vi "Tektonik.vi"() -> ()   [LabVIEW 2015]
uses:
  <vilib>/Utility/error.llb/DialogType.ctl
  <instrlib>/Tektronix TDS 200 1000 2000 Series/Public/Data/Read (Single Waveform).vi
  <vilib>/express/express analysis/Spectral/Block/exnSpectralBlock spectral measurements RMS poly.vi
  <vilib>/express/express analysis/Spectral/Block/exnSpectralBlock spectral measurements RMS WFM.vi
  <vilib>/express/express analysis/Spectral/XNode/ExpressSpectralMeasurementsBlockNode.xnode
  <instrlib>/Tektronix TDS 200 1000 2000 Series/Tektronix TDS 200 1000 2000 Series.lvlib
panel:
  out "Units 2":string
  out "Vpp":dbl
  out "FFT":cluster{"f0":dbl, "df":dbl, "magnitude":dbl[]}(graph)
  out "Units":string
  out "Freq":dbl
  in  "VISA resource name":refnum<visa-resource-name>
  in  "Serial Configuration":T1={"Baud Rate"=9600, "Parity"=0, "Stop Bits"=10, "Flow Control"=2} {"Flow Control" items=["None", "XON/XOFF", "RTS/CTS", "XON/XOFF & RTS/CTS", "DTR/DSR", "XON/XOFF & DTR/DSR"]; "Stop Bits" items=["1.0"=10, "1.5"=15, "2.0"=20]; "Parity" items=["None", "Odd", "Even", "Mark", "Space"]; "Baud Rate" items=["300"=300, "600"=600, "1200"=1200, "2400"=2400, "4800"=4800, "9600"=9600, "19200"=19200]}
  out "Waveform Graph":waveform(dbl)(graph)
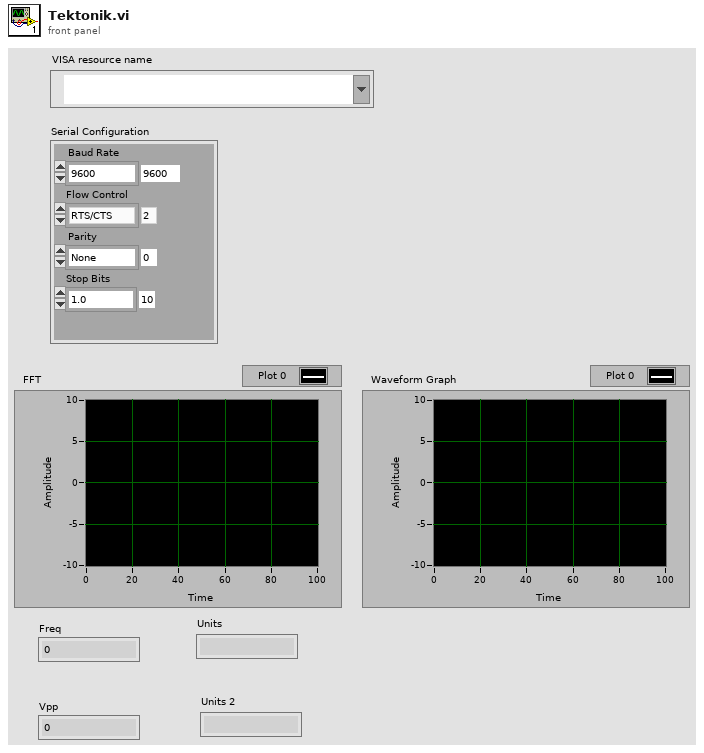
[diagram p1: front panel]
types:
  T1 = cluster{"Baud Rate":u32, "Parity":u16, "Stop Bits":u16, "Flow Control":u16}
  T2 = typedef "DialogType.ctl" = u16
  T3 = cluster{"averaging mode":u16, "weighting mode":u16, "number of averages":u32}
  T4 = cluster{"dB On (F)":bool, "unwrap phase (F)":bool, "convert to degree (F)":bool}
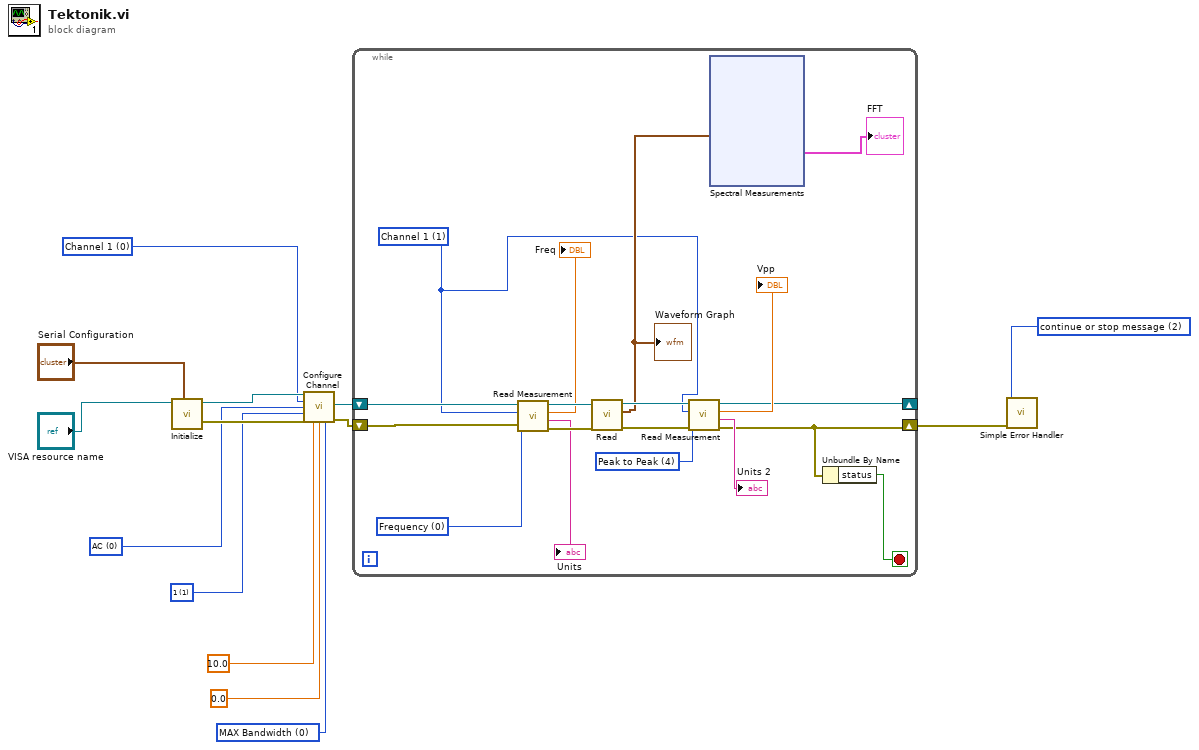
[diagram p0: block diagram]
diagram:
  w1 = T2 2 items=["no dialog", "OK message", "continue or stop message", "OK message + warnings", "continue/stop + warnings"] ("type of dialog (OK msg:1)")
  w2 = 0 items=["MAX Bandwidth", "Unlimited"] ("Bandwidth (0: MAX Bandwidth)")
  w5 = 1 items=["1"=1, "10"=10, "20"=20, "50"=50, "100"=100, "500"=500, "1000"=1000] ("Probe Attenuation (10: 10X)")
  w6 = 0 items=["AC", "DC", "Ground"] ("Vertical Coupling (1: DC)")
  w7 = 0 items=["Channel 1", "Channel 2", "Channel 3", "Channel 4", "Math", "Reference A", "Reference B", "Reference C", "Reference D"] ("Channel (0: Channel 1)")
  n1 = call <instrlib>:"Initialize.vi"("Serial Configuration"="Serial Configuration", "VISA resource name"="VISA resource name") -> ("error out"=w11:errorcluster, "VISA resource name out"=w8:refnum<visa-resource-name>)  [unwired: 8 in]
  n2 = call <instrlib>:"Configure Channel.vi"("VISA resource name"=w8, "Channel (0: Channel 1)"=w7, "Vertical Coupling (1: DC)"=w6, "Probe Attenuation (10: 10X)"=w5, "error in (no error)"=w11, "Vertical Range (10.0 V/div)"=10.0, "Vertical Offset (0.0 divs)"=0.0, "Bandwidth (0: MAX Bandwidth)"=w2) -> ("VISA resource name out"=w9:refnum<visa-resource-name>, "error out"=w10:errorcluster)  [unwired: 6 in]
  n3 = while {
    shift-right: [w15] -> w14
    shift-left: w10 -> [w30]
    shift-right: [w16] -> _
    shift-left: w9 -> [w29]
    stop <- w17 stop-if-true
    w21 = 4 items=["Frequency", "Mean", "Period", "Pulse Duty", "Peak to Peak", "Cycle RMS", "Minimum", "Maximum", "Rise Time", "Fall Time", "Positive Width", "Negative Width", "Amplitude", "Cycle Mean", "High", "Low", "Negative Duty", "Positive Overshoot", "Negative Overshoot", "Cursor Mean", "Burst Width", "Positive Pulse Count", "Negative Pulse Count", "Rising Edge Count", "Falling Edge Count", "Area", "Cycle Area", "RMS", "Cursor RMS"] ("Measurement Type (0: Frequency)")
    w26 = 0 items=["Frequency", "Mean", "Period", "Pulse Duty", "Peak to Peak", "Cycle RMS", "Minimum", "Maximum", "Rise Time", "Fall Time", "Positive Width", "Negative Width", "Amplitude", "Cycle Mean", "High", "Low", "Negative Duty", "Positive Overshoot", "Negative Overshoot", "Cursor Mean", "Burst Width", "Positive Pulse Count", "Negative Pulse Count", "Rising Edge Count", "Falling Edge Count", "Area", "Cycle Area", "RMS", "Cursor RMS"] ("Measurement Type (0: Frequency)")
    w20 = 1 items=["Channel 1"=1, "Channel 2"=2, "Channel 3"=3, "Channel 4"=4] ("Channel (1: Channel 1)")
    n4 = call <instrlib>:"Read Measurement.vi"("error in (no error)"=w30, "Measurement Type (0: Frequency)"=w26, "Channel (1: Channel 1)"=w20, "VISA resource name"=w29) -> ("error out"=w32:errorcluster, "Units"=→"Units":string, "Measurement"=→"Freq":dbl, "VISA resource name out"=w28:refnum<visa-resource-name>)  [unwired: 4 in]
    n5 = call-poly <instrlib>:"Read.vi"("error in (no error)"=w32, "VISA resource name"=w28) -> ("error out"=w31:errorcluster, "Waveform Data"=w23:waveform(dbl), "VISA resource name out"=w27:refnum<visa-resource-name>)  [unwired: 7 in]
    "Waveform Graph" <- w23
    n6 = call <instrlib>:"Read Measurement.vi"("error in (no error)"=w31, "Measurement Type (0: Frequency)"=w21, "Channel (1: Channel 1)"=w20, "VISA resource name"=w27) -> ("error out"=w15:errorcluster, "Units"=→"Units 2":string, "Measurement"=→"Vpp":dbl, "VISA resource name out"=w16:refnum<visa-resource-name>)  [unwired: 4 in]
    n7 = xnode "Spectral Measurements"("Signals"=w23) -> ("FFT - (RMS)"=→"FFT":cluster{"f0":dbl, "df":dbl, "magnitude":dbl[]})  [unwired: 1 in, 2 out]
    n8 = Unbundle By Name(w15) -> ("status"=w17:bool)
  }
  n9 = call <vilib>:"Simple Error Handler.vi"("type of dialog (OK msg:1)"=w1, "error in (no error)"=w14) -> ()  [unwired: 3 in, 5 out]
